vi "Merge Data.vi"(8 "error in":errorcluster, 10 "Analyzed":refnum<class "Instrument.lvclass">, 11 "Acquired":refnum<class "PAS.lvclass">) -> (0 "error out":errorcluster, 3 "PAS out":refnum<class "PAS.lvclass">)   [LabVIEW 2015, in "PAS.lvclass"]
doc: "Merge the analyzed data with that of the current retrieved data set. In this case, we are only concerned with insuring that the cell quality and resonant frequency are properly populated."
uses:
  PAS.lvclass
  Instrument/Instrument.lvclass
  PAS.lvclass/PAS.ctl
  Data/Cell/PAS Cell Data.lvclass/PAS Cell Data.ctl
  Data/Cell/Read IAbackground.vi
  Data/Cell/Write IAbackground.vi
  Data/Read measTime.vi
  Data/Cell/Read derived.vi
  Data/Cell/Read freqData.vi
  Data/Cell/Read lasDiodeData.vi
  Data/Cell/Write derived.vi
  File IO/Class/File Observer.lvclass
  Data/Main/PAS Data.lvclass
  Data/Cell/PAS Cell Data.lvclass
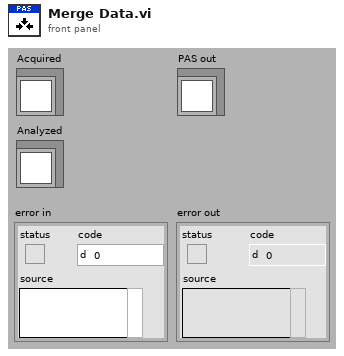
[diagram p1: front panel]
types:
  T1 = cluster{"f0":sgl, "IA":sgl, "Q":sgl, "max":dbl[], "deltaPhi":dbl, "tau":dbl, "noiseLim":dbl, "ext":dbl}
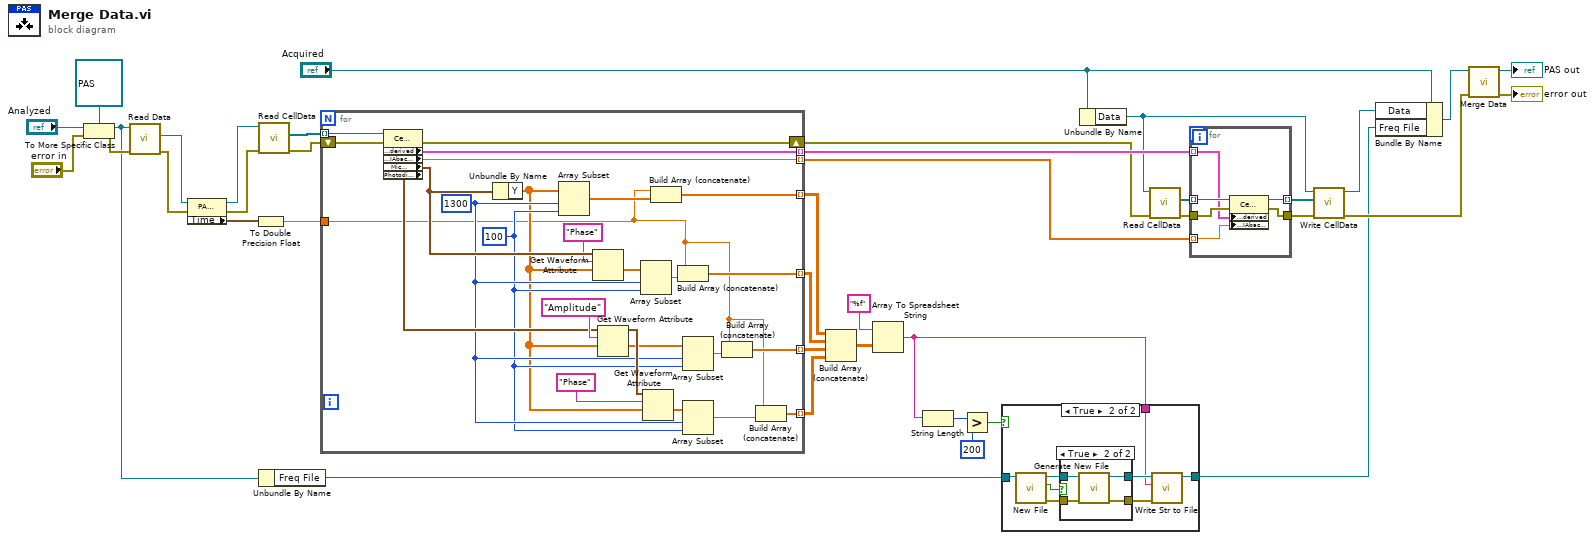
[diagram p0: block diagram]
diagram:
  n1 = To More Specific Class(target class=refnum<class "PAS.lvclass"> refnum ("PAS in"), reference="Analyzed", error in="error in") -> (specific class reference=w20:refnum<class "PAS.lvclass">, error out=w29:errorcluster)
  n2 = call "Read Data.vi"("error in"=w29, "PAS in"=w20) -> ("error out"=w16:errorcluster, "PAS Data.lvclass"=w18:refnum<class "PAS Data.lvclass">)  [unwired: 7 in, 1 out]
  n3 = property class="PAS Data"(reference=w18, error in=w16) -> (reference out=w17:refnum<class "PAS Data.lvclass">, error out=w15:errorcluster, "Time"=w14:timestamp)
  n4 = To Double Precision Float(number=w14) -> (double precision float=w13:dbl)
  n5 = call "Read CellData.vi"("error in"=w15, "PAS Data in"=w17) -> ("error out"=w34:errorcluster, "CellData"=w35:refnum<class "PAS Cell Data.lvclass">[])  [unwired: 7 in, 1 out]
  n6 = Unbundle By Name(w20) -> ("Freq File"=w19:refnum<class "File Observer.lvclass">)
  n7 = for {
    tunnel: w35 -> [w65] mode=indexing
    tunnel: [w64] -> w33 mode=indexing
    tunnel: [w62] -> w22 mode=indexing
    tunnel: w13 -> [w41]
    tunnel: [w60] -> w10 mode=indexing
    tunnel: [w47] -> w9 mode=indexing
    tunnel: [w40] -> w3 mode=indexing
    tunnel: [w44] -> w2 mode=indexing
    shift-right: [w63] -> w1
    shift-left: w34 -> [w50]
    w52 = 100 ("length")
    w53 = 1300 ("index")
    n8 = property class="Cell Data"(reference=w65, error in=w50) -> (error out=w63:errorcluster, "Data Access:derived"=w64:T1, "Data Access:IAbackground"=w62:dbl, "Mic Frequency"=w59:waveform(sgl), "Photodiode"=w55:waveform(i16))  [unwired: 1 out]
    n9 = Unbundle By Name(w59) -> ("Y"=w51:sgl[])
    n10 = Array Subset(array=w51, index=w53, length=w52) -> (w61:sgl[])
    n11 = Get Waveform Attribute(5:w51, 6:"Phase" ("name"), 7:w59) -> (1:w48:sgl[])  [unwired: 1 in, 3 out]
    n12 = Get Waveform Attribute(5:w51, 6:"Amplitude" ("name"), 7:w55) -> (1:w46:sgl[], 3:w54:waveform(i16))  [unwired: 1 in, 2 out]
    n13 = Array Subset(array=w48, index=w53, length=w52) -> (w49:sgl[])
    n14 = Get Waveform Attribute(5:w51, 6:"Phase" ("name"), 7:w54) -> (1:w42:sgl[])  [unwired: 1 in, 3 out]
    n15 = Build Array (concatenate)(w41, w61) -> (w60:dbl[])
    n16 = Build Array (concatenate)(w41, w49) -> (w47:dbl[])
    n17 = Array Subset(array=w46, index=w53, length=w52) -> (w45:sgl[])
    n18 = Array Subset(array=w42, index=w53, length=w52) -> (w43:sgl[])
    n19 = Build Array (concatenate)(w41, w45) -> (w44:dbl[])
    n20 = Build Array (concatenate)(w41, w43) -> (w40:dbl[])
  }
  n21 = Build Array (concatenate)(w10, w9, w2, w3) -> (w8:dbl[][])
  n22 = Array To Spreadsheet String(array=w8, 3:"%f" ("format string")) -> (spreadsheet string=w7:string)  [unwired: 1 in]
  n23 = String Length(string=w7) -> (length=w6:i32)
  n24 = Greater?(x=w6, y=200) -> (0:w4:bool)
  n25 = case shown="True" w4 {
    tunnel: w19 -> [w66 w74]
    tunnel: [w66 w68] -> w11
    tunnel: w7 -> [_ w67]
    frame False {
    }
    frame True {
      n26 = call-dynamic "New File.vi"("File Observer in"=w74) -> ("error out"=w71:errorcluster, "Exceeded"=w73:bool, "File Observer out"=w72:refnum<class "File Observer.lvclass">)  [unwired: 8 in]
      n27 = case shown="True" w73 {
        tunnel: w72 -> [w76 w80]
        tunnel: [w76 w79] -> w70
        tunnel: w71 -> [w75 w78]
        tunnel: [w75 w77] -> w69
        frame False {
        }
        frame True {
          n28 = call-dynamic "Generate New File.vi"("error in"=w78, "File Obs in"=w80) -> ("error out"=w77:errorcluster, "File Obs out"=w79:refnum<class "File Observer.lvclass">)  [unwired: 7 in, 1 out]
        }
      }
      n29 = call "Write Str to File.vi"("error in"=w69, "Str to Write"=w67, "File Obs in"=w70) -> ("File Obs out"=w68:refnum<class "File Observer.lvclass">)  [unwired: 7 in, 1 out]
    }
  }
  n30 = Unbundle By Name("Acquired") -> ("Data"=w26:refnum<class "PAS Data.lvclass">)
  n31 = call "Read CellData.vi"("error in"=w1, "PAS Data in"=w26) -> ("error out"=w38:errorcluster, "CellData"=w36:refnum<class "PAS Cell Data.lvclass">[])  [unwired: 7 in, 1 out]
  n32 = for {
    tunnel: w36 -> [w86] mode=indexing
    tunnel: [w83] -> w37 mode=indexing
    tunnel: w38 -> [w85]
    tunnel: [w84] -> w39
    tunnel: w33 -> [w82] mode=indexing
    tunnel: w22 -> [w81] mode=indexing
    n33 = property class="Cell Data"(reference=w86, error in=w85, "Data Access:derived"=w82, "Data Access:IAbackground"=w81) -> (reference out=w83:refnum<class "PAS Cell Data.lvclass">, error out=w84:errorcluster)
  }
  n34 = call "Write CellData.vi"("error in"=w39, "CellData"=w37, "PAS Data in"=w26) -> ("error out"=w23:errorcluster, "PAS Data out"=w25:refnum<class "PAS Data.lvclass">)  [unwired: 7 in]
  n35 = Bundle By Name(cluster="Acquired", "Data"=w25, "Freq File"=w11) -> (w24:refnum<class "PAS.lvclass">)
  n36 = call-parent "Merge Data.vi"("error in"=w23, "Acquired"=w24) -> ("error out"=→"error out":errorcluster, "Instrument out"=→"PAS out":refnum<class "PAS.lvclass">)  [unwired: 8 in]
